vi "Get Time.vi"(8 "error in (no error)":errorcluster, 11 "CIFCorePlugin in":refnum<class "CIFCorePlugin.lvclass">) -> (0 "error out":errorcluster, 2 "Time (ns)":u64, 3 "CIFCorePlugin out":refnum<class "CIFCorePlugin.lvclass">)   [LabVIEW 2021, in "CIFCorePlugin.lvclass"]
uses:
  CIFCorePlugin.lvclass
  CIFUtilities/CIFClocks/Time Conversion/LabVIEW Time to UTC Time.vi
  CIFUtilities/CIFClocks/SubVIs/Add Error.vi
  CIFUtilities/CIFClocks/CIFClocks.lvlib
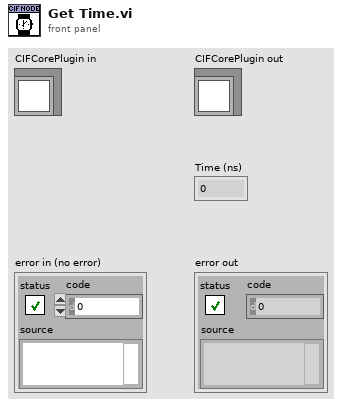
[diagram p1: front panel]
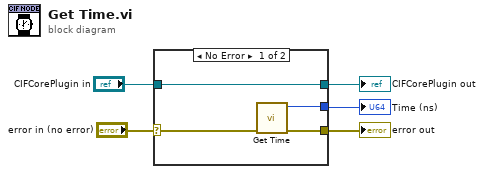
[diagram p0: block diagram]
diagram:
  n1 = case shown="No Error" "error in (no error)" {
    selector: "error in (no error)" -> [w6 w10]
    tunnel: [w8 w10] -> w4
    tunnel: [w7 w11] -> w2
    tunnel: "CIFCorePlugin in" -> [w7 w11]
    tunnel: [w9 _] -> w1
    frame No Error {
      n2 = call "Get Time.vi"("error in (no error)"=w6) -> ("error out"=w8:errorcluster, "Time (ns)"=w9:u64)  [unwired: 8 in, 1 out]
    }
    frame Error {
    }
  }
  "error out" <- w4
  "CIFCorePlugin out" <- w2
  "Time (ns)" <- w1
